vi "Connect.vi"(0 "Axis":string, 1 "VISA resource name":refnum<visa-resource-name>, 2 "baud rate (9600)":u32=9600, 3 "Controller #":u8=1, 4 "Joystick buttons":T1={"MinDir"=1, "MaxDir"=2, "MedSpeed"=5, "HighSpeed"=6} {"HighSpeed" min=1 max=25 step=1; "MedSpeed" min=1 max=25 step=1; "MaxDir" min=1 max=25 step=1; "MinDir" min=1 max=25 step=1}, 5 "error in":errorcluster) -> (14 "Zaber":T2={"Serial port handle"="", "Axis"="", "Controller #"=0, "Min position"=0.0, "Max position"=0.0, "Min velocity"=0.0, "Max velocity"=0.0, "Firmware"="", "Device ID"=0, "Variable event"=refnum, "Variable ref"=refnum, "Resolution, usteps/step"=0, "Serial port semaphore"=refnum, "Joystick buttons"={"MinDir"=1, "MaxDir"=2, "MedSpeed"=5, "HighSpeed"=6}} {"Joystick buttons"."HighSpeed" min=1 max=25 step=1; "Joystick buttons"."MedSpeed" min=1 max=25 step=1; "Joystick buttons"."MaxDir" min=1 max=25 step=1; "Joystick buttons"."MinDir" min=1 max=25 step=1}, 19 "error out":errorcluster)   [LabVIEW 2018]
uses:
  Zaber.ctl
  GenericDataEvent/GenericEvent.ctl
  ZaberVariables.ctl
  Stage joystick buttons.ctl
  GenericDataEvent/GenericData.ctl
  <vilib>/Instr/_visa.llb/VISA Configure Serial Port (Instr).vi
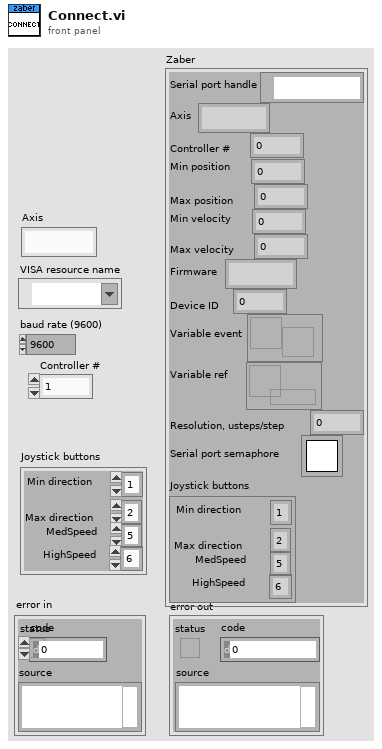
[diagram p1: front panel]
types:
  T1 = typedef "Stage joystick buttons.ctl" = cluster{"MinDir":i32, "MaxDir":i32, "MedSpeed":i32, "HighSpeed":i32}
  T2 = typedef "Zaber.ctl" = cluster{"Serial port handle":refnum<visa-resource-name>, "Axis":string, "Controller #":u8, "Min position":dbl, "Max position":dbl, "Min velocity":dbl, "Max velocity":dbl, "Firmware":string, "Device ID":i32, "Variable event":T3, "Variable ref":refnum<data-value>, "Resolution, usteps/step":i32, "Serial port semaphore":T4, "Joystick buttons":cluster{"MinDir":i32, "MaxDir":i32, "MedSpeed":i32, "HighSpeed":i32}}
  T3 = typedef "GenericEvent.ctl" = refnum<user-event>
  T4 = typedef "Semaphore RefNum" = refnum<k1>
  T5 = typedef "ZaberVariables.ctl" = cluster{"Position":i32, "Speed":i32, "Min soft position":dbl, "Max soft position":dbl, "Accelaration":i32}
  T6 = typedef "GenericData.ctl" = cluster{"Name":string, "Data":variant}
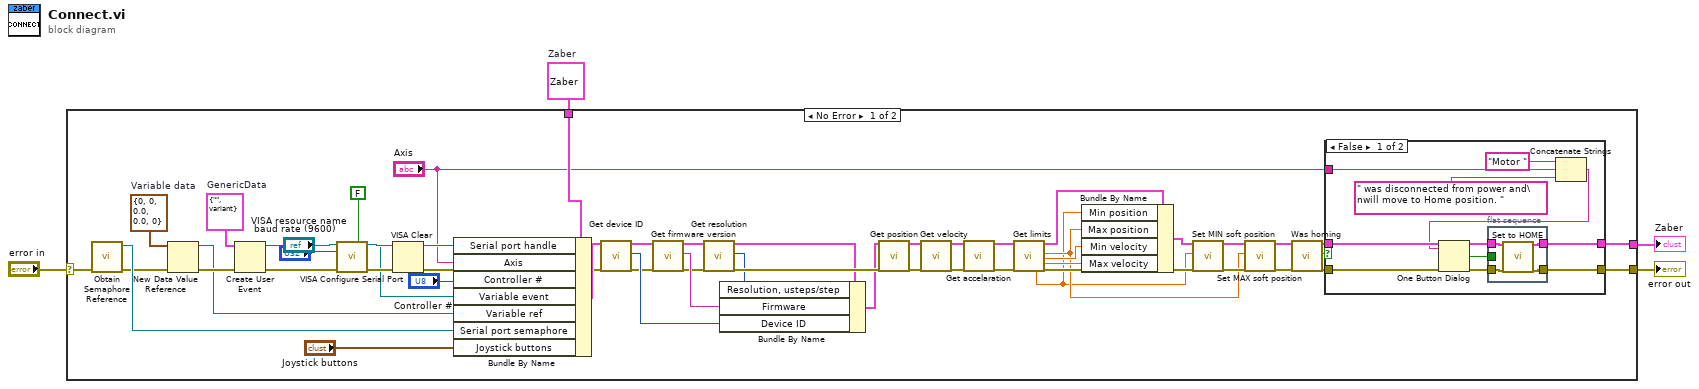
[diagram p0: block diagram]
diagram:
  w3 = T2 {"Serial port handle"="", "Axis"="", "Controller #"=0, "Min position"=0.0, "Max position"=0.0, "Min velocity"=0.0, "Max velocity"=0.0, "Firmware"="", "Device ID"=0, "Variable event"=refnum, "Variable ref"=refnum, "Resolution, usteps/step"=0, "Serial port semaphore"=refnum, "Joystick buttons"={"MinDir"=1, "MaxDir"=2, "MedSpeed"=5, "HighSpeed"=6}}  # Zaber
  n1 = case shown="No Error" "error in" {
    selector: "error in" -> [w17 w74]
    tunnel: [w28 w74] -> w1
    tunnel: [w29 w73] -> w2
    tunnel: w3 -> [w57 w73]
    frame No Error {
      w7 = T5 {"Position"=0, "Speed"=0, "Min soft position"=0.0, "Max soft position"=0.0, "Accelaration"=0}  # Variable data
      w41 = T6 {"Name"="", "Data"=variant}  # GenericData
      n2 = call <vilib>:"Obtain Semaphore Reference.vi"("error in (no error)"=w17) -> ("error out"=w16:errorcluster, "semaphore"=w18:T4)  [unwired: 4 in, 1 out]
      n3 = New Data Value Reference(data value=w7, error in=w16) -> (data value reference=w34:refnum<data-value>, error out=w36:errorcluster)
      n4 = Create User Event(user event datatype=w41, error in=w36) -> (user event=w42:refnum<user-event>, error out=w35:errorcluster)
      n5 = call-poly "VISA Configure Serial Port"("VISA resource name"="VISA resource name", "Enable Termination\nChar (T)"=FALSE ("Enable Termination\nChar (T)"), "baud rate (9600)"="baud rate (9600)", "error in (no error)"=w35) -> ("VISA resource name out"=w55:refnum<visa-resource-name>, "error out"=w56:errorcluster)  [unwired: 10 in]
      n6 = VISA Clear(VISA resource name=w55, error in (no error)=w56) -> (VISA resource name out=w53:refnum<visa-resource-name>, error out=w37:errorcluster)
      n7 = Bundle By Name(cluster=w57, "Serial port handle"=w53, "Axis"="Axis", "Controller #"="Controller #", "Variable event"=w42, "Variable ref"=w34, "Serial port semaphore"=w18, "Joystick buttons"="Joystick buttons") -> (w44:T2)
      n8 = call "Get device ID.vi"("Zaber"=w44, "error in"=w37) -> ("Zaber out"=w24:T2, "Device ID"=w26:i32, "error out"=w25:errorcluster)  [unwired: 15 in]
      n9 = call "Get firmware version.vi"("Zaber"=w24, "error in"=w25) -> ("Zaber out"=w21:T2, "Firmware version"=w27:string, "error out"=w23:errorcluster)  [unwired: 15 in]
      n10 = call "Get resolution.vi"("Zaber in"=w21, "error in"=w23) -> ("Zaber out"=w20:T2, "Resolution, usteps/step"=w19:u16, "error out"=w22:errorcluster)  [unwired: 15 in]
      n11 = Bundle By Name(cluster=w20, "Resolution, usteps/step"=w19, "Firmware"=w27, "Device ID"=w26) -> (w15:T2)
      n12 = call "Get position.vi"("Zaber"=w15, "error in"=w22) -> ("Zaber out"=w38:T2, "error out"=w39:errorcluster)  [unwired: 13 in, 3 out]
      n13 = call "Get velocity.vi"("Zaber"=w38, "error in"=w39) -> ("Zaber out"=w31:T2, "error out"=w33:errorcluster)  [unwired: 14 in, 2 out]
      n14 = call "Get accelaration.vi"("Zaber"=w31, "error in"=w33) -> ("Zaber out"=w30:T2, "error out"=w32:errorcluster)  [unwired: 14 in, 2 out]
      n15 = call "Get limits.vi"("Zaber"=w30, "error in"=w32) -> ("MIN position, mm"=w6:dbl, "Zaber out"=w49:T2, "MAX position, mm"=w8:dbl, "MIN velociry, mm/s"=w48:dbl, "MAX velocity, mm/s"=w43:dbl, "error out"=w13:errorcluster)  [unwired: 11 in, 1 out]
      n16 = Bundle By Name(cluster=w49, "Min position"=w6, "Max position"=w8, "Min velocity"=w48, "Max velocity"=w43) -> (w12:T2)
      n17 = call "Set MIN soft position.vi"("Zaber"=w12, "Min soft position"=w6, "error in"=w13) -> ("Zaber out"=w11:T2, "error out"=w14:errorcluster)  [unwired: 14 in, 1 out]
      n18 = call "Set MAX soft position.vi"("Zaber"=w11, "Max soft position"=w8, "error in"=w14) -> ("Zaber out"=w10:T2, "error out"=w9:errorcluster)  [unwired: 14 in, 1 out]
      n19 = call "Was homing.vi"("Zaber"=w10, "error in"=w9) -> ("Zaber out"=w45:T2, "Was homing?"=w47:bool, "error out"=w46:errorcluster)  [unwired: 15 in]
      n20 = case shown="False" w47 {
        tunnel: w46 -> [w65 w71]
        tunnel: [w64 w71] -> w28
        tunnel: w45 -> [w63 w72]
        tunnel: [w62 w72] -> w29
        tunnel: "Axis" -> [w59 _]
        frame False {
          n21 = flat-sequence {
            tunnel: w66 -> [_]
            tunnel: w65 -> [w70]
            tunnel: [w69] -> w64
            tunnel: w63 -> [w68]
            tunnel: [w67] -> w62
            frame #0 {
              n22 = call "Set to HOME.vi"("Zaber"=w68, "error in"=w70) -> ("Zaber out"=w67:T2, "error out"=w69:errorcluster)  [unwired: 16 in]
            }
          }
          n23 = Concatenate Strings("Motor " ("string"), w59, " was disconnected from power and\nwill move to Home position. " ("message")) -> (w58:string)
          n24 = One Button Dialog(message=w58) -> (true=w66:bool)  [unwired: 1 in]
        }
        frame True {
        }
      }
    }
    frame Error {
    }
  }
  "error out" <- w1
  "Zaber" <- w2
